vi "Wrap Angle And Calculate Components.vi"(11 "Angle in [deg]":sgl) -> (3 "Angle out [deg]":sgl)   [LabVIEW 2015, in "Math.lvlib"]
uses:
  Math.lvlib
  <vilib>/Analysis/coordinate.llb/Angle Units.ctl
  <vilib>/Analysis/coordinate.llb/Angle Range (Degree).ctl
  <vilib>/Analysis/coordinate.llb/Wrap Angle (scalar).vi
  <vilib>/Analysis/NI_AAL_Angle.lvlib
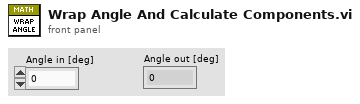
[diagram p1: front panel]
types:
  T1 = typedef "NI_AAL_Angle.lvlib/Angle Range (Degree).ctl" = u16
  T2 = typedef "NI_AAL_Angle.lvlib/Angle Units.ctl" = i32
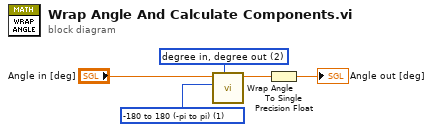
[diagram p0: block diagram]
diagram:
  w3 = T1 1 items=["none", "-180 to 180 (-pi to pi)", "0 to 360 (0 to 2pi)"] ("angle range")
  w2 = T2 2 items=["radian in, radian out", "radian in, degree out", "degree in, degree out", "degree in, radian out"] ("angle units")
  n1 = call-poly <vilib>:"Wrap Angle.vi"("angle units"=w2, "angle range"=w3, "angle in"="Angle in [deg]") -> ("angle out"=w4:dbl)  [unwired: 7 in, 1 out]
  n2 = To Single Precision Float(number=w4) -> (single precision float=→"Angle out [deg]":sgl)
